vi "Show-hide controls.vi"(8 "Error In":errorcluster, 10 "Multimetro":T1, 11 "Data In":T2) -> (0 "Error Out":errorcluster, 3 "Data Out":T2)   [LabVIEW 2015]
doc: "VI used to show/hide controls of each type of measurements depending on what multimeter is selected."
uses:
  controls/UI Data.ctl
  controls/Instruments.ctl
  <vilib>/Utility/miscctls.llb/LVPositionTypeDef.ctl
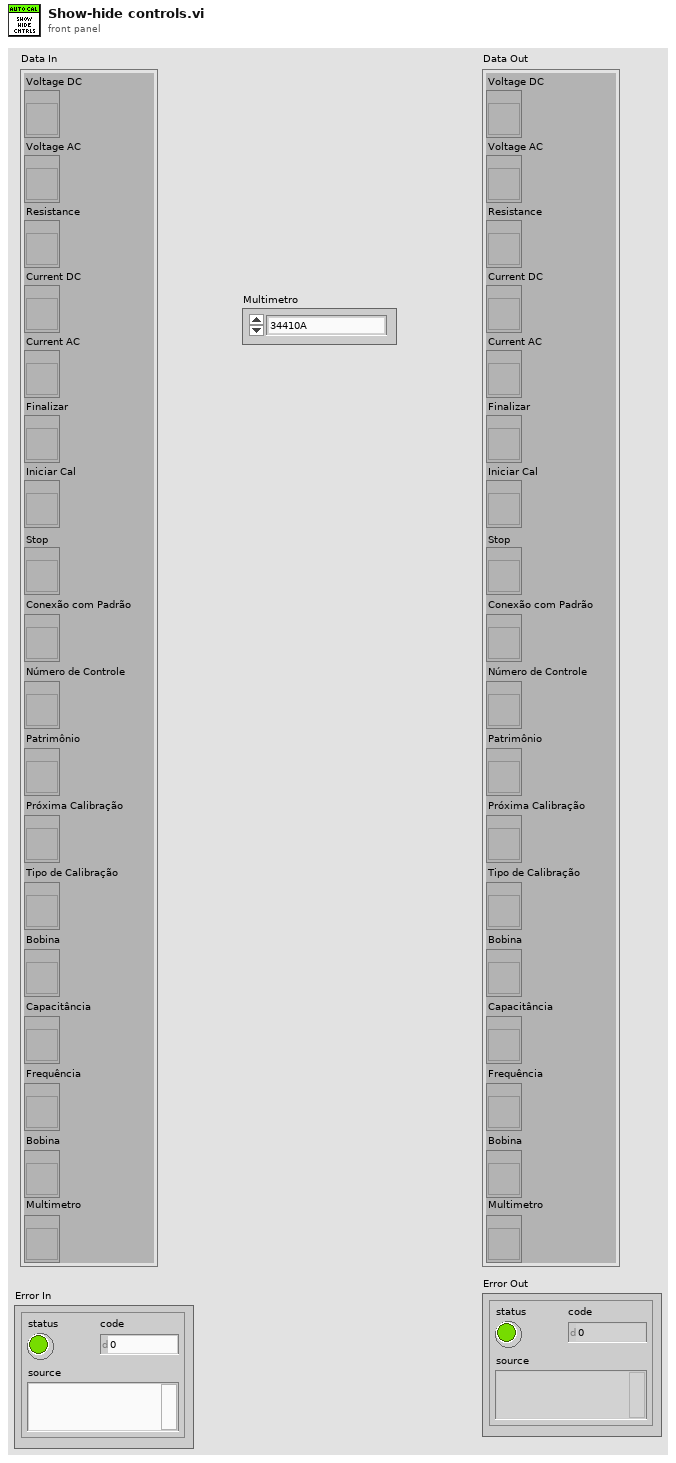
[diagram p1: front panel]
types:
  T1 = typedef "Instruments.ctl" = enum16{"34410A", "34401A", "U1252B", "U1252A", "U1213A", "8845A", "8846A", "189", "289", "DMM4050", "TY720"}
  T2 = typedef "UI Data.ctl" = cluster{"Voltage DC":refnum<vi>, "Voltage AC":refnum<vi>, "Resistance":refnum<vi>, "Current DC":refnum<vi>, "Current AC":refnum<vi>, "Finalizar":refnum<vi>, "Iniciar Cal":refnum<vi>, "Stop":refnum<vi>, "Conexão com Padrão":refnum<vi>, "Número de Controle":refnum<vi>, "Patrimônio":refnum<vi>, "Próxima Calibração":refnum<vi>, "Tipo de Calibração":refnum<vi>, "Bobina":refnum<vi>, "Capacitância":refnum<vi>, "Frequência":refnum<vi>, "Bobina":refnum<vi>, "Multimetro":refnum<vi>}
  T3 = typedef "LVPositionTypeDef.ctl" = cluster{"Left":i32, "Top":i32}
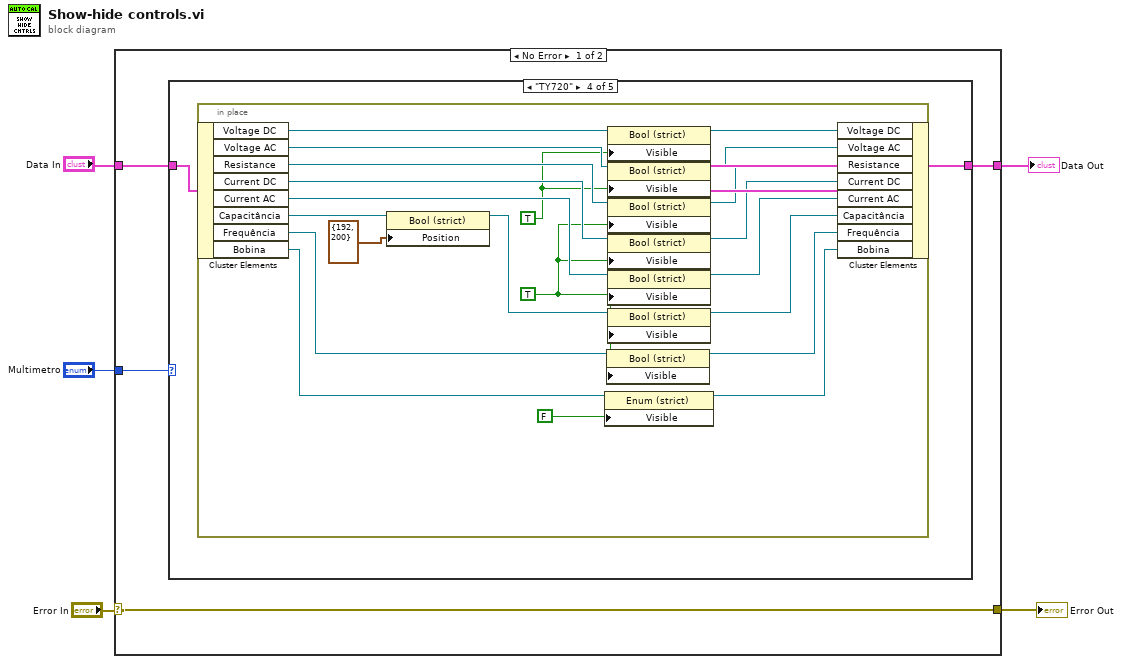
[diagram p0: block diagram]
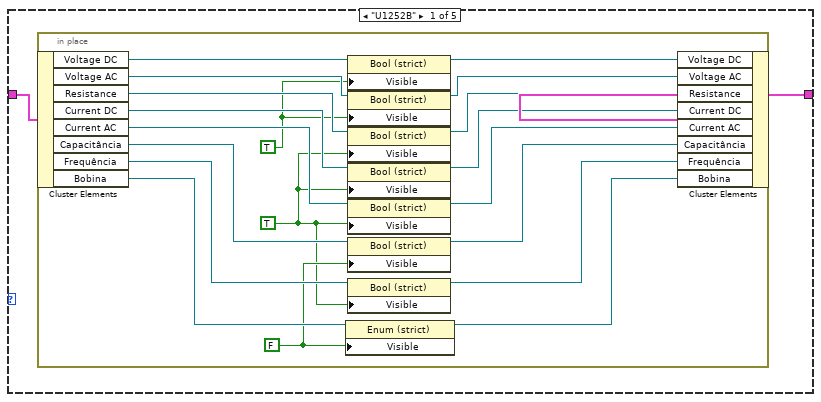
[diagram p2: hidden frame]
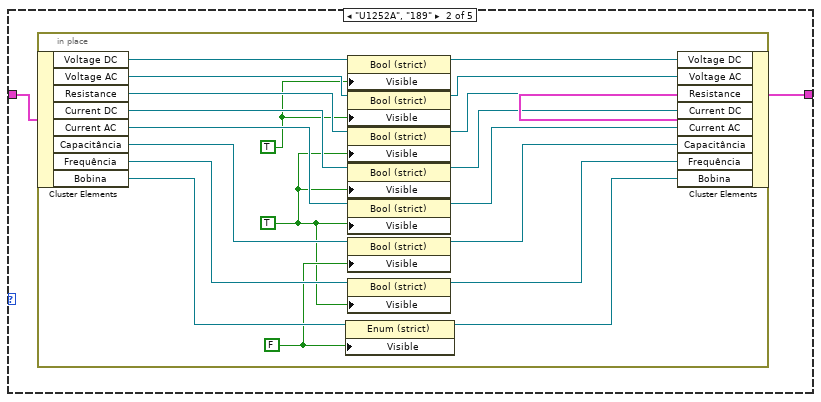
[diagram p3: hidden frame]
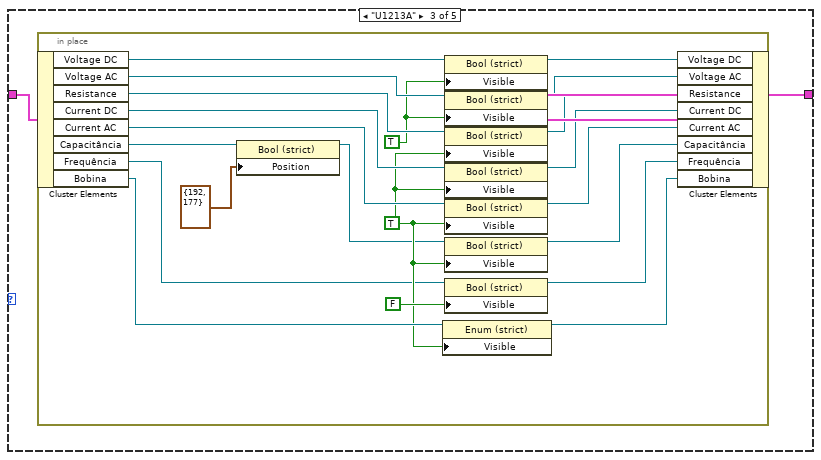
[diagram p4: hidden frame]
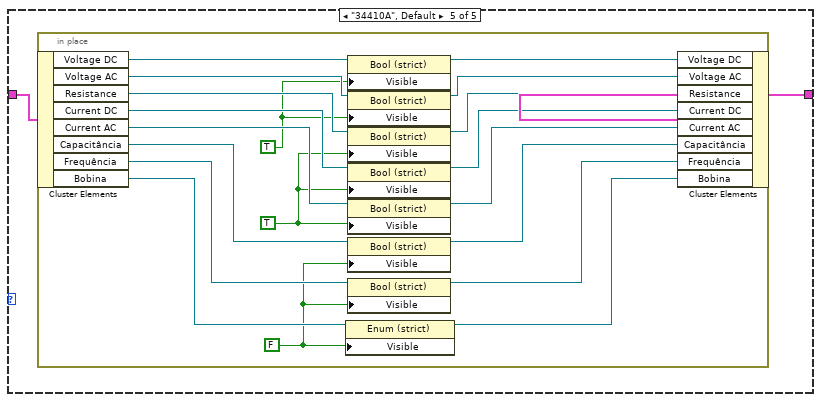
[diagram p5: hidden frame]
diagram:
  n1 = case shown="No Error" "Error In" {
    selector: "Error In" -> [w6 w120]
    tunnel: "Data In" -> [w9 w119]
    tunnel: [w8 w119] -> w4
    tunnel: "Multimetro" -> [w7 _]
    tunnel: [w6 w120] -> w1
    frame No Error {
      n2 = case shown="\"TY720\"" w7 {
        tunnel: w9 -> [w11 w32 w53 w76 w99]
        tunnel: [w10 w31 w52 w75 w98] -> w8
        frame "U1252B" {
          n3 = in-place {
            w13 = FALSE
            w20 = TRUE
            w12 = TRUE
            n4 = in-place-cluster #1(w11) -> ("Voltage DC"=w30:refnum<vi>, "Voltage AC"=w29:refnum<vi>, "Resistance"=w28:refnum<vi>, "Current DC"=w27:refnum<vi>, "Current AC"=w26:refnum<vi>, "Capacitância"=w19:refnum<vi>, "Frequência"=w18:refnum<vi>, "Bobina"=w17:refnum<vi>)
            n5 = property class="Enum (strict)"(reference=w17, "Visible"=w13) -> (reference out=w16:refnum<vi>)  [unwired: 1 in, 1 out]
            n6 = property class="Bool (strict)"(reference=w30, "Visible"=w20) -> (reference out=w25:refnum<vi>)  [unwired: 1 in, 1 out]
            n7 = property class="Bool (strict)"(reference=w29, "Visible"=w20) -> (reference out=w24:refnum<vi>)  [unwired: 1 in, 1 out]
            n8 = property class="Bool (strict)"(reference=w28, "Visible"=w12) -> (reference out=w23:refnum<vi>)  [unwired: 1 in, 1 out]
            n9 = property class="Bool (strict)"(reference=w27, "Visible"=w12) -> (reference out=w22:refnum<vi>)  [unwired: 1 in, 1 out]
            n10 = property class="Bool (strict)"(reference=w26, "Visible"=w12) -> (reference out=w21:refnum<vi>)  [unwired: 1 in, 1 out]
            n11 = property class="Bool (strict)"(reference=w19, "Visible"=w13) -> (reference out=w14:refnum<vi>)  [unwired: 1 in, 1 out]
            n12 = property class="Bool (strict)"(reference=w18, "Visible"=w12) -> (reference out=w15:refnum<vi>)  [unwired: 1 in, 1 out]
            n13 = in-place-cluster #1("Voltage DC"=w25, "Voltage AC"=w24, "Resistance"=w23, "Current DC"=w22, "Current AC"=w21, "Capacitância"=w14, "Frequência"=w15, "Bobina"=w16) -> (w10:T2)
          }
        }
        frame "U1252A", "189" {
          n14 = in-place {
            w34 = FALSE
            w41 = TRUE
            w33 = TRUE
            n15 = in-place-cluster #2(w32) -> ("Voltage DC"=w51:refnum<vi>, "Voltage AC"=w50:refnum<vi>, "Resistance"=w49:refnum<vi>, "Current DC"=w48:refnum<vi>, "Current AC"=w47:refnum<vi>, "Capacitância"=w40:refnum<vi>, "Frequência"=w39:refnum<vi>, "Bobina"=w38:refnum<vi>)
            n16 = property class="Enum (strict)"(reference=w38, "Visible"=w34) -> (reference out=w37:refnum<vi>)  [unwired: 1 in, 1 out]
            n17 = property class="Bool (strict)"(reference=w51, "Visible"=w41) -> (reference out=w46:refnum<vi>)  [unwired: 1 in, 1 out]
            n18 = property class="Bool (strict)"(reference=w50, "Visible"=w41) -> (reference out=w45:refnum<vi>)  [unwired: 1 in, 1 out]
            n19 = property class="Bool (strict)"(reference=w49, "Visible"=w33) -> (reference out=w44:refnum<vi>)  [unwired: 1 in, 1 out]
            n20 = property class="Bool (strict)"(reference=w48, "Visible"=w33) -> (reference out=w43:refnum<vi>)  [unwired: 1 in, 1 out]
            n21 = property class="Bool (strict)"(reference=w47, "Visible"=w33) -> (reference out=w42:refnum<vi>)  [unwired: 1 in, 1 out]
            n22 = property class="Bool (strict)"(reference=w40, "Visible"=w34) -> (reference out=w35:refnum<vi>)  [unwired: 1 in, 1 out]
            n23 = property class="Bool (strict)"(reference=w39, "Visible"=w33) -> (reference out=w36:refnum<vi>)  [unwired: 1 in, 1 out]
            n24 = in-place-cluster #2("Voltage DC"=w46, "Voltage AC"=w45, "Resistance"=w44, "Current DC"=w43, "Current AC"=w42, "Capacitância"=w35, "Frequência"=w36, "Bobina"=w37) -> (w31:T2)
          }
        }
        frame "U1213A" {
          n25 = in-place {
            w64 = TRUE
            w58 = TRUE
            n26 = in-place-cluster #3(w53) -> ("Voltage DC"=w74:refnum<vi>, "Voltage AC"=w73:refnum<vi>, "Resistance"=w72:refnum<vi>, "Current DC"=w71:refnum<vi>, "Current AC"=w70:refnum<vi>, "Capacitância"=w56:refnum<vi>, "Frequência"=w57:refnum<vi>, "Bobina"=w63:refnum<vi>)
            n27 = property class="Bool (strict)"(reference=w56, "Position"=T3 {"Left"=192, "Top"=177} ("Caption.Position 2")) -> (reference out=w54:refnum<vi>)  [unwired: 1 in, 1 out]
            n28 = property class="Enum (strict)"(reference=w63, "Visible"=w58) -> (reference out=w62:refnum<vi>)  [unwired: 1 in, 1 out]
            n29 = property class="Bool (strict)"(reference=w74, "Visible"=w64) -> (reference out=w69:refnum<vi>)  [unwired: 1 in, 1 out]
            n30 = property class="Bool (strict)"(reference=w73, "Visible"=w64) -> (reference out=w68:refnum<vi>)  [unwired: 1 in, 1 out]
            n31 = property class="Bool (strict)"(reference=w72, "Visible"=w58) -> (reference out=w67:refnum<vi>)  [unwired: 1 in, 1 out]
            n32 = property class="Bool (strict)"(reference=w71, "Visible"=w58) -> (reference out=w66:refnum<vi>)  [unwired: 1 in, 1 out]
            n33 = property class="Bool (strict)"(reference=w70, "Visible"=w58) -> (reference out=w65:refnum<vi>)  [unwired: 1 in, 1 out]
            n34 = property class="Bool (strict)"(reference=w54, "Visible"=w58) -> (reference out=w60:refnum<vi>)  [unwired: 1 in, 1 out]
            n35 = property class="Bool (strict)"(reference=w57, "Visible"=FALSE) -> (reference out=w61:refnum<vi>)  [unwired: 1 in, 1 out]
            n36 = in-place-cluster #3("Voltage DC"=w69, "Voltage AC"=w68, "Resistance"=w67, "Current DC"=w66, "Current AC"=w65, "Capacitância"=w60, "Frequência"=w61, "Bobina"=w62) -> (w52:T2)
          }
        }
        frame "TY720" {
          n37 = in-place {
            w87 = TRUE
            w80 = TRUE
            n38 = in-place-cluster #4(w76) -> ("Voltage DC"=w97:refnum<vi>, "Voltage AC"=w96:refnum<vi>, "Resistance"=w95:refnum<vi>, "Current DC"=w94:refnum<vi>, "Current AC"=w93:refnum<vi>, "Capacitância"=w78:refnum<vi>, "Frequência"=w86:refnum<vi>, "Bobina"=w85:refnum<vi>)
            n39 = property class="Bool (strict)"(reference=w78, "Position"=T3 {"Left"=192, "Top"=200} ("Caption.Position")) -> (reference out=w79:refnum<vi>)  [unwired: 1 in, 1 out]
            n40 = property class="Enum (strict)"(reference=w85, "Visible"=FALSE) -> (reference out=w84:refnum<vi>)  [unwired: 1 in, 1 out]
            n41 = property class="Bool (strict)"(reference=w86, "Visible"=w80) -> (reference out=w83:refnum<vi>)  [unwired: 1 in, 1 out]
            n42 = property class="Bool (strict)"(reference=w97, "Visible"=w87) -> (reference out=w92:refnum<vi>)  [unwired: 1 in, 1 out]
            n43 = property class="Bool (strict)"(reference=w96, "Visible"=w87) -> (reference out=w91:refnum<vi>)  [unwired: 1 in, 1 out]
            n44 = property class="Bool (strict)"(reference=w95, "Visible"=w80) -> (reference out=w90:refnum<vi>)  [unwired: 1 in, 1 out]
            n45 = property class="Bool (strict)"(reference=w94, "Visible"=w80) -> (reference out=w89:refnum<vi>)  [unwired: 1 in, 1 out]
            n46 = property class="Bool (strict)"(reference=w93, "Visible"=w80) -> (reference out=w88:refnum<vi>)  [unwired: 1 in, 1 out]
            n47 = property class="Bool (strict)"(reference=w79, "Visible"=w80) -> (reference out=w82:refnum<vi>)  [unwired: 1 in, 1 out]
            n48 = in-place-cluster #4("Voltage DC"=w92, "Voltage AC"=w91, "Resistance"=w90, "Current DC"=w89, "Current AC"=w88, "Capacitância"=w82, "Frequência"=w83, "Bobina"=w84) -> (w75:T2)
          }
        }
        frame "34410A", Default {
          n49 = in-place {
            w100 = FALSE
            w108 = TRUE
            w101 = TRUE
            n50 = in-place-cluster #5(w99) -> ("Voltage DC"=w118:refnum<vi>, "Voltage AC"=w117:refnum<vi>, "Resistance"=w116:refnum<vi>, "Current DC"=w115:refnum<vi>, "Current AC"=w114:refnum<vi>, "Capacitância"=w107:refnum<vi>, "Frequência"=w106:refnum<vi>, "Bobina"=w105:refnum<vi>)
            n51 = property class="Enum (strict)"(reference=w105, "Visible"=w100) -> (reference out=w104:refnum<vi>)  [unwired: 1 in, 1 out]
            n52 = property class="Bool (strict)"(reference=w118, "Visible"=w108) -> (reference out=w113:refnum<vi>)  [unwired: 1 in, 1 out]
            n53 = property class="Bool (strict)"(reference=w117, "Visible"=w108) -> (reference out=w112:refnum<vi>)  [unwired: 1 in, 1 out]
            n54 = property class="Bool (strict)"(reference=w116, "Visible"=w101) -> (reference out=w111:refnum<vi>)  [unwired: 1 in, 1 out]
            n55 = property class="Bool (strict)"(reference=w115, "Visible"=w101) -> (reference out=w110:refnum<vi>)  [unwired: 1 in, 1 out]
            n56 = property class="Bool (strict)"(reference=w114, "Visible"=w101) -> (reference out=w109:refnum<vi>)  [unwired: 1 in, 1 out]
            n57 = property class="Bool (strict)"(reference=w107, "Visible"=w100) -> (reference out=w102:refnum<vi>)  [unwired: 1 in, 1 out]
            n58 = property class="Bool (strict)"(reference=w106, "Visible"=w100) -> (reference out=w103:refnum<vi>)  [unwired: 1 in, 1 out]
            n59 = in-place-cluster #5("Voltage DC"=w113, "Voltage AC"=w112, "Resistance"=w111, "Current DC"=w110, "Current AC"=w109, "Capacitância"=w102, "Frequência"=w103, "Bobina"=w104) -> (w98:T2)
          }
        }
      }
    }
    frame Error {
    }
  }
  "Data Out" <- w4
  "Error Out" <- w1
